vi "Initiate Model and Serial Numbers.vi"(6 "Measurement Role Selection":T1, 7 "UI Device Type":T2, 8 "error in (no error)":errorcluster, 9 "Serial CmbBox Ref":refnum<vi>, 10 "Model CmbBox Ref":refnum<vi>, 11 "Database in":refnum<queue>) -> (0 "error out":errorcluster, 3 "Database out":refnum<queue>)   [LabVIEW 2026, in "Settings.lvlib"]
uses:
  Settings.lvlib
  support/Architecture/Message Queue/Message Cluster.ctl
  controls/UI/Data Entity.ctl
  controls/UI/Measurement Role Selection.ctl
  controls/UI/UI List Type.ctl
  support/Architecture/Message Queue/Message Queue.lvlib
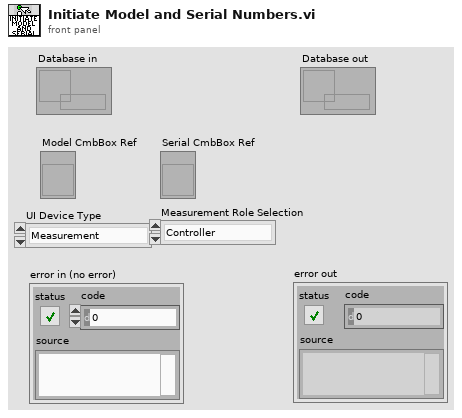
[diagram p1: front panel]
types:
  T1 = typedef "Settings.lvlib/Measurement Role Selection.ctl" = enum16{"Controller", "Reference", "UUT", "All"}
  T2 = typedef "Settings.lvlib/Data Entity.ctl" = enum16{"Measurement", "Controller", " Test Configuration"}
  T3 = typedef "UI List Type.ctl" = enum16{"Model Numbers", "Serial Numbers", "Operators", "Calibration Points", "Start Run Times"}
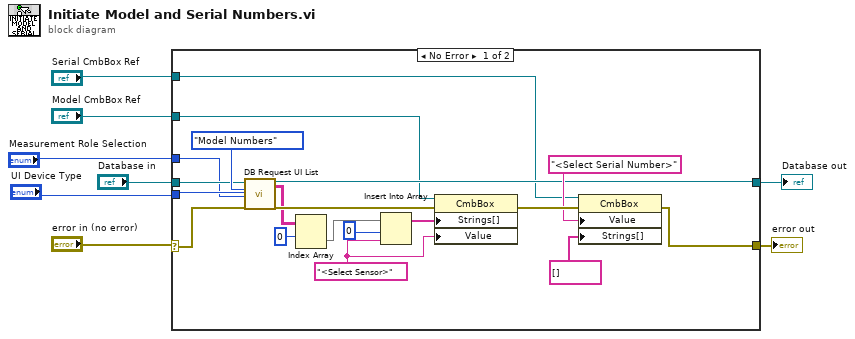
[diagram p0: block diagram]
diagram:
  n1 = case shown="No Error" "error in (no error)" {
    selector: "error in (no error)" -> [w15 w29]
    tunnel: [w13 w29] -> w8
    tunnel: "Database in" -> [w19 w28]
    tunnel: [w18 w28] -> w6
    tunnel: "Serial CmbBox Ref" -> [w17 _]
    tunnel: "Model CmbBox Ref" -> [w16 _]
    tunnel: "UI Device Type" -> [w14 _]
    tunnel: "Measurement Role Selection" -> [w9 _]
    frame No Error {
      w25 = "<Select Sensor>"
      n2 = call "DB Request UI List.vi"("Database in"=w19, "UI List Type"=UI_List_Type."Model Numbers", "UI Device Type"=w14, "Measurement Role Selection"=w9, "error in (no error)"=w15) -> ("Database out"=w18:refnum<queue>, "Results"=w12:string[][], "error out"=w23:errorcluster)  [unwired: 12 in]
      n3 = Index Array(array=w12, index (row)=0) -> (element=w10:string[])  [unwired: 1 in]
      n4 = Insert Into Array(array=w10, index=0, new element=w25) -> (w26:string[])
      n5 = property on="Property Node" class="CmbBox"(reference=w16, error in=w23, "Strings[]"=w26, "Value"=w25) -> (error out=w27:errorcluster)  [unwired: 1 out]
      n6 = property on="Property Node" class="CmbBox"(reference=w17, error in=w27, "Value"="<Select Serial Number>", "Strings[]"=string[] [] ("Strings []")) -> (error out=w13:errorcluster)  [unwired: 1 out]
    }
    frame Error {
    }
  }
  "error out" <- w8
  "Database out" <- w6
